vi "MB_TCP_7016_p.vi"(6 "N":i32, 9 "timeouts":T1={"conn_timeout"=1000, "reconn_timeout"=3000, "N attempt max"=3, "t_reset_TTL"=120000, "write_timeout"=10, "read_timeout"=500, "period"=100} {"t_reset_TTL" min=10 max=240000 step=1; "period" min=10 max=100000 step=1; "read_timeout" min=10 max=60000 step=1; "write_timeout" min=1 max=60000 step=1; "N attempt max" min=1 max=5 step=1; "reconn_timeout" min=10 max=240000 step=1; "conn_timeout" min=10 max=240000}, 10 "write enable":bool=TRUE, 11 "stop":bool) -> (0 "error out":errorcluster, 2 "errors":u32, 3 "Z3":u32)   [LabVIEW 2019]
uses:
  NI_modbus_upd/NI_modbus_upd.lvlib
  NI_modbus_upd.llb/MB Modbus Command.ctl
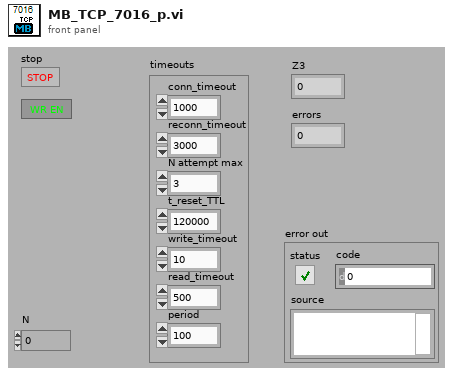
[diagram p1: front panel]
types:
  T1 = cluster{"conn_timeout":i32, "reconn_timeout":u32, "N attempt max":i32, "t_reset_TTL":u32, "write_timeout":i32, "read_timeout":i32, "period":u32}
  T2 = enum16{"Init", "Read", "Read inputs", "Read outputs", "Write", "Write inputs"}
  T3 = enum16{"DI", "DO to write", "DO", "AI", "AO to write", "AO", "DI AI", "DI AO", "DO AI", "DO AO"}
  T4 = enum16{"Start", "Connect", "Write enable", "IP address", "Errors"}
  T5 = typedef "MB Modbus Command.ctl" = cluster{"Function Code":u8, "Starting Address":u16, "Quantity":u16, "Data":u16[], "Discrete":bool[]}
  T6 = cluster{"Transaction ID":u16, "Protocol ID":u16, "Length":u16, "Unit ID":u8}
  T7 = cluster{"Remote IP Address":string, "Remote Port":u16}
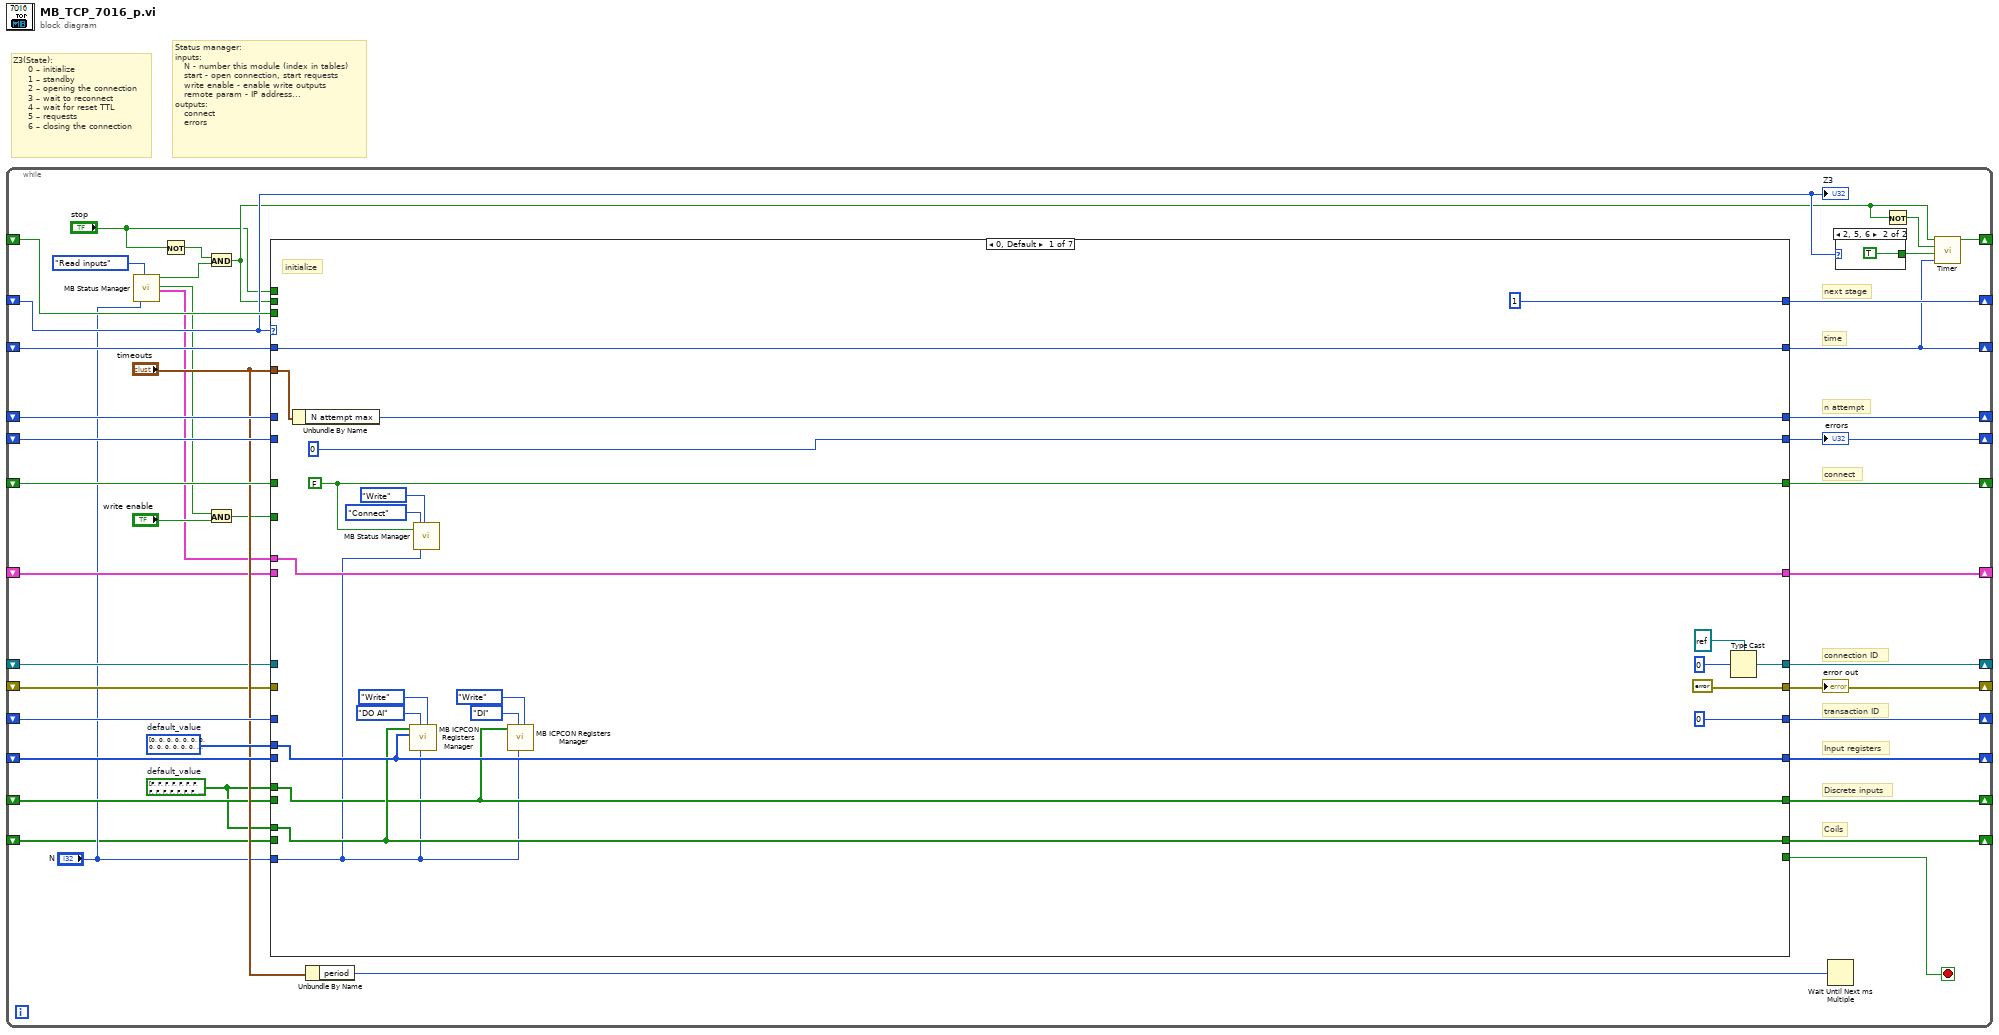
[diagram p0: block diagram]
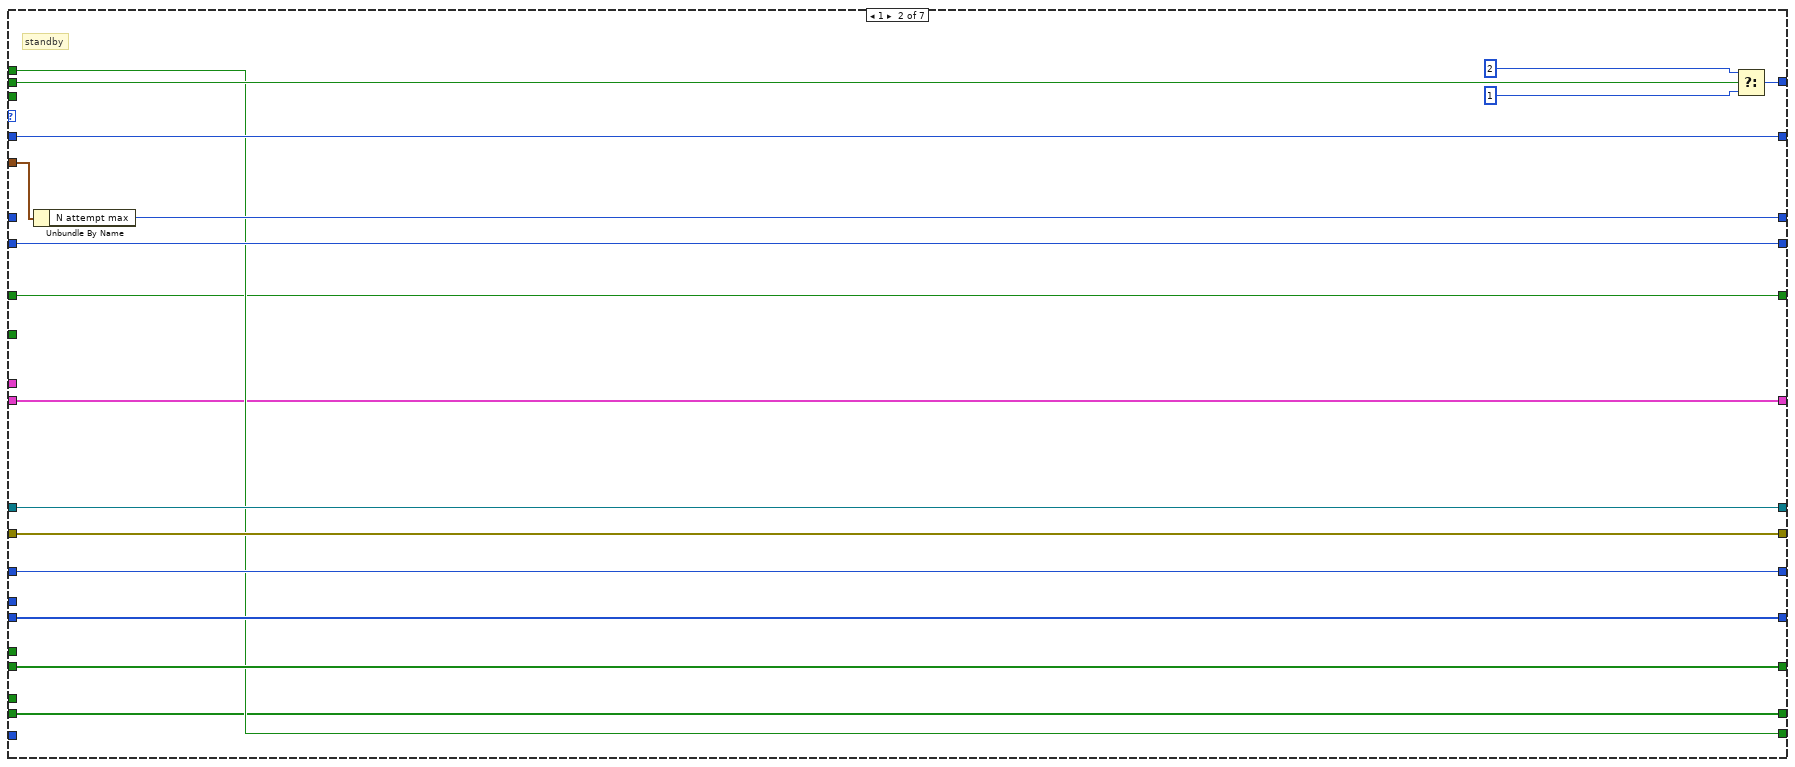
[diagram p2: hidden frame]
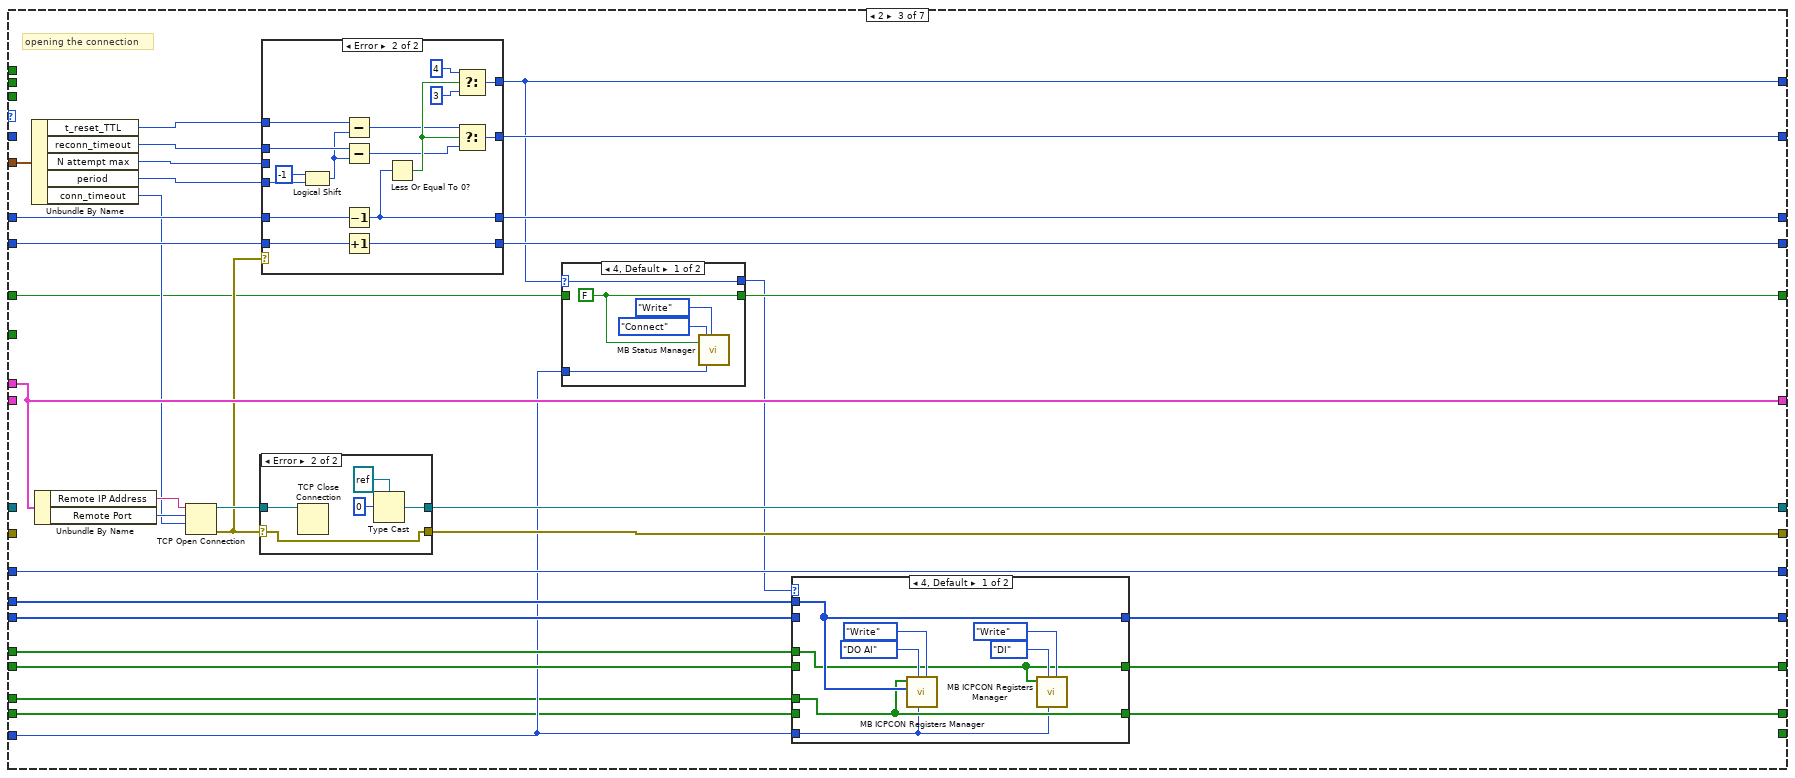
[diagram p3: hidden frame]
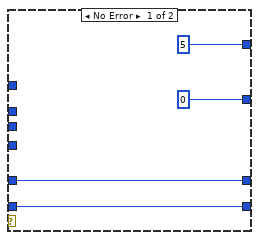
[diagram p7: hidden frame]
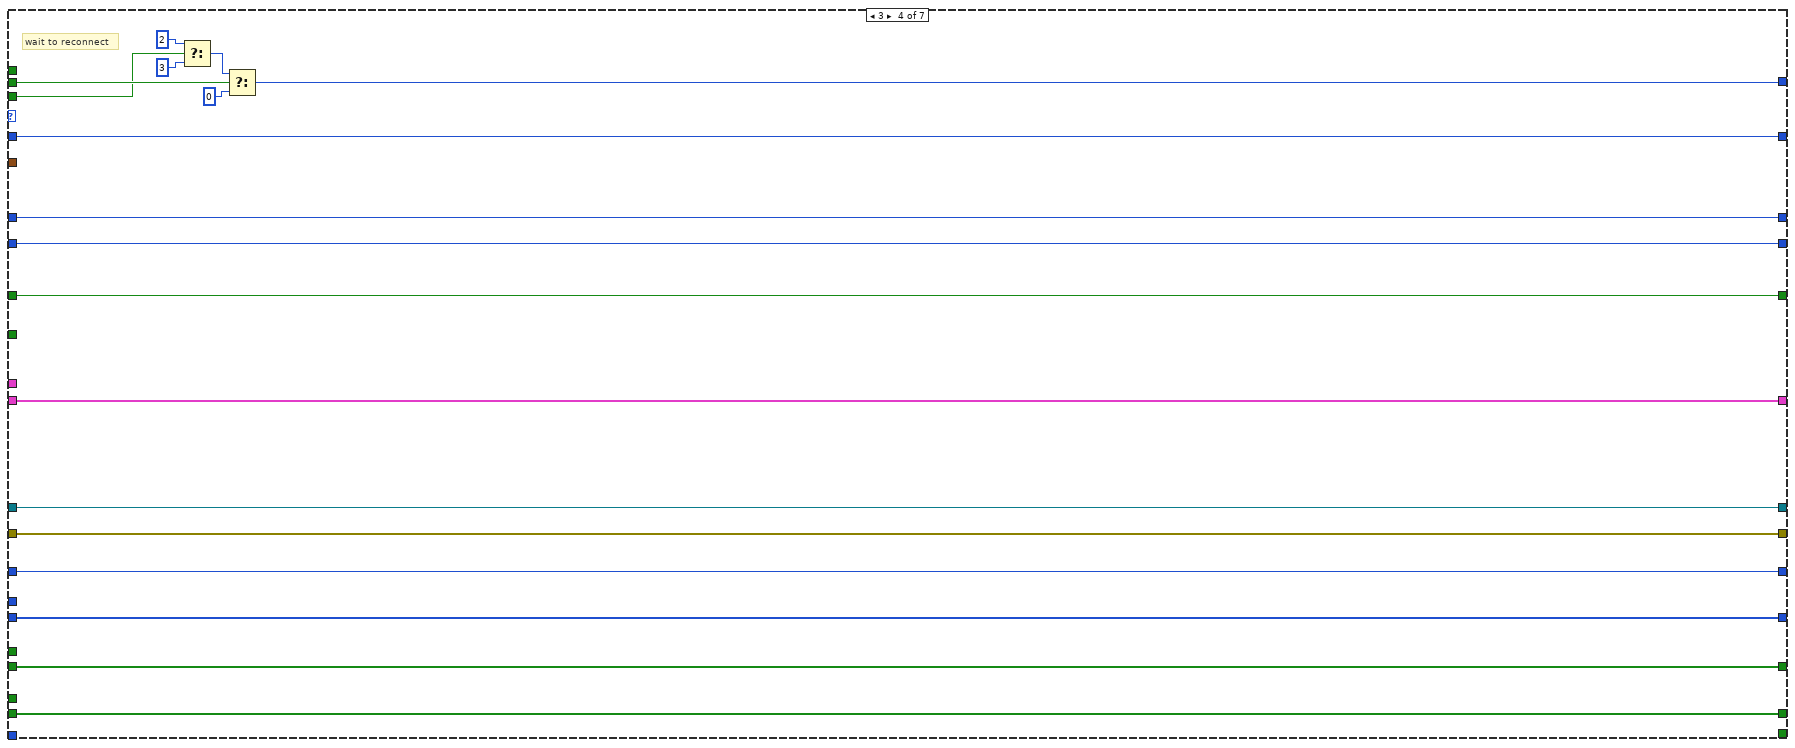
[diagram p8: hidden frame]
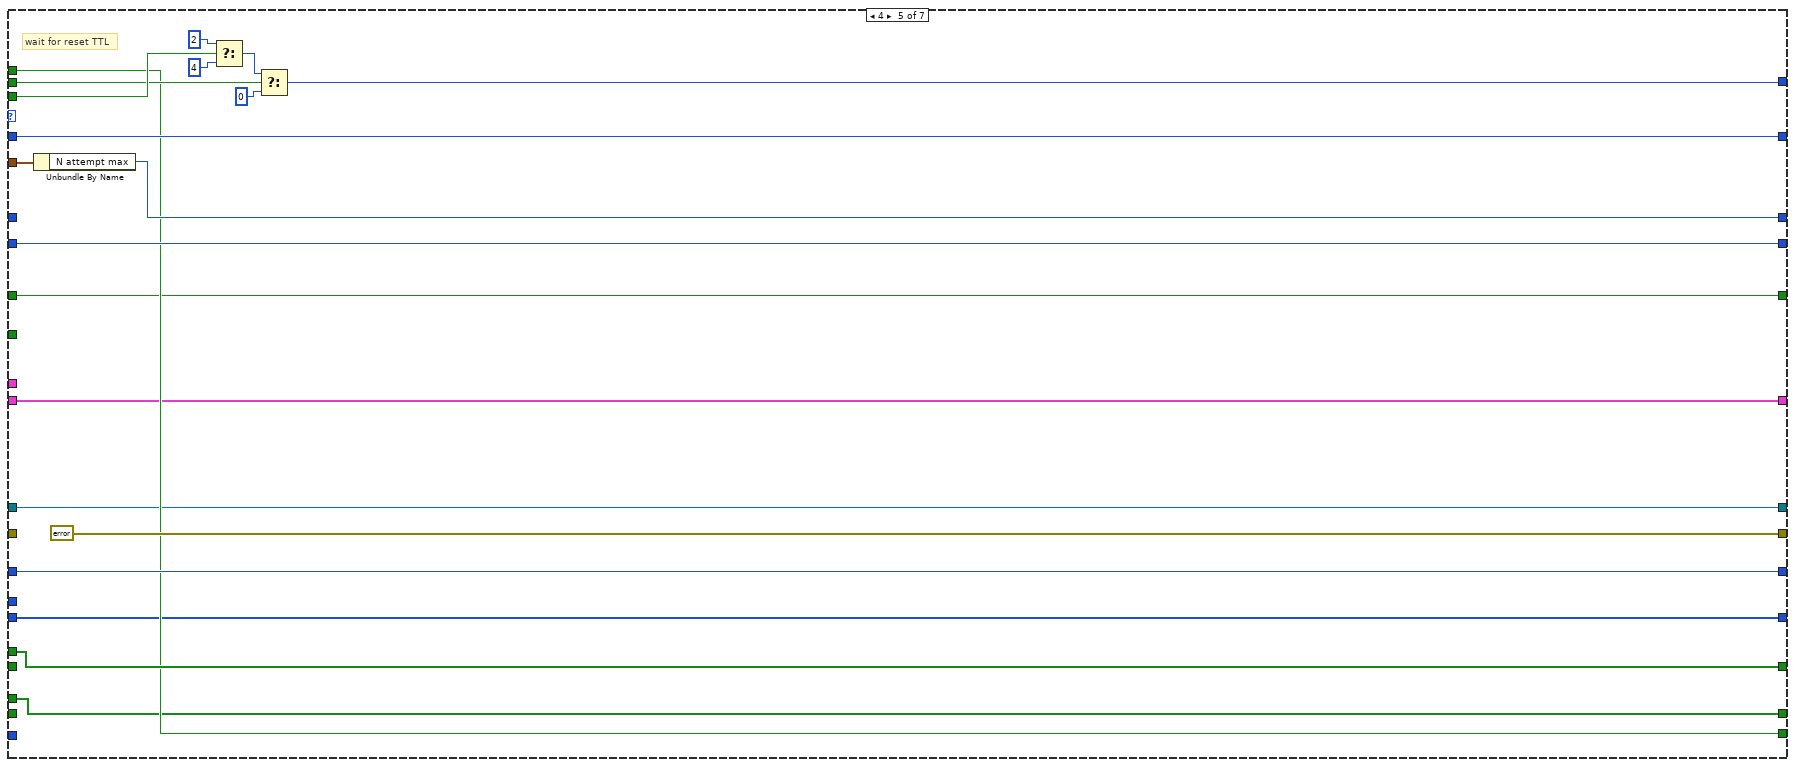
[diagram p9: hidden frame]
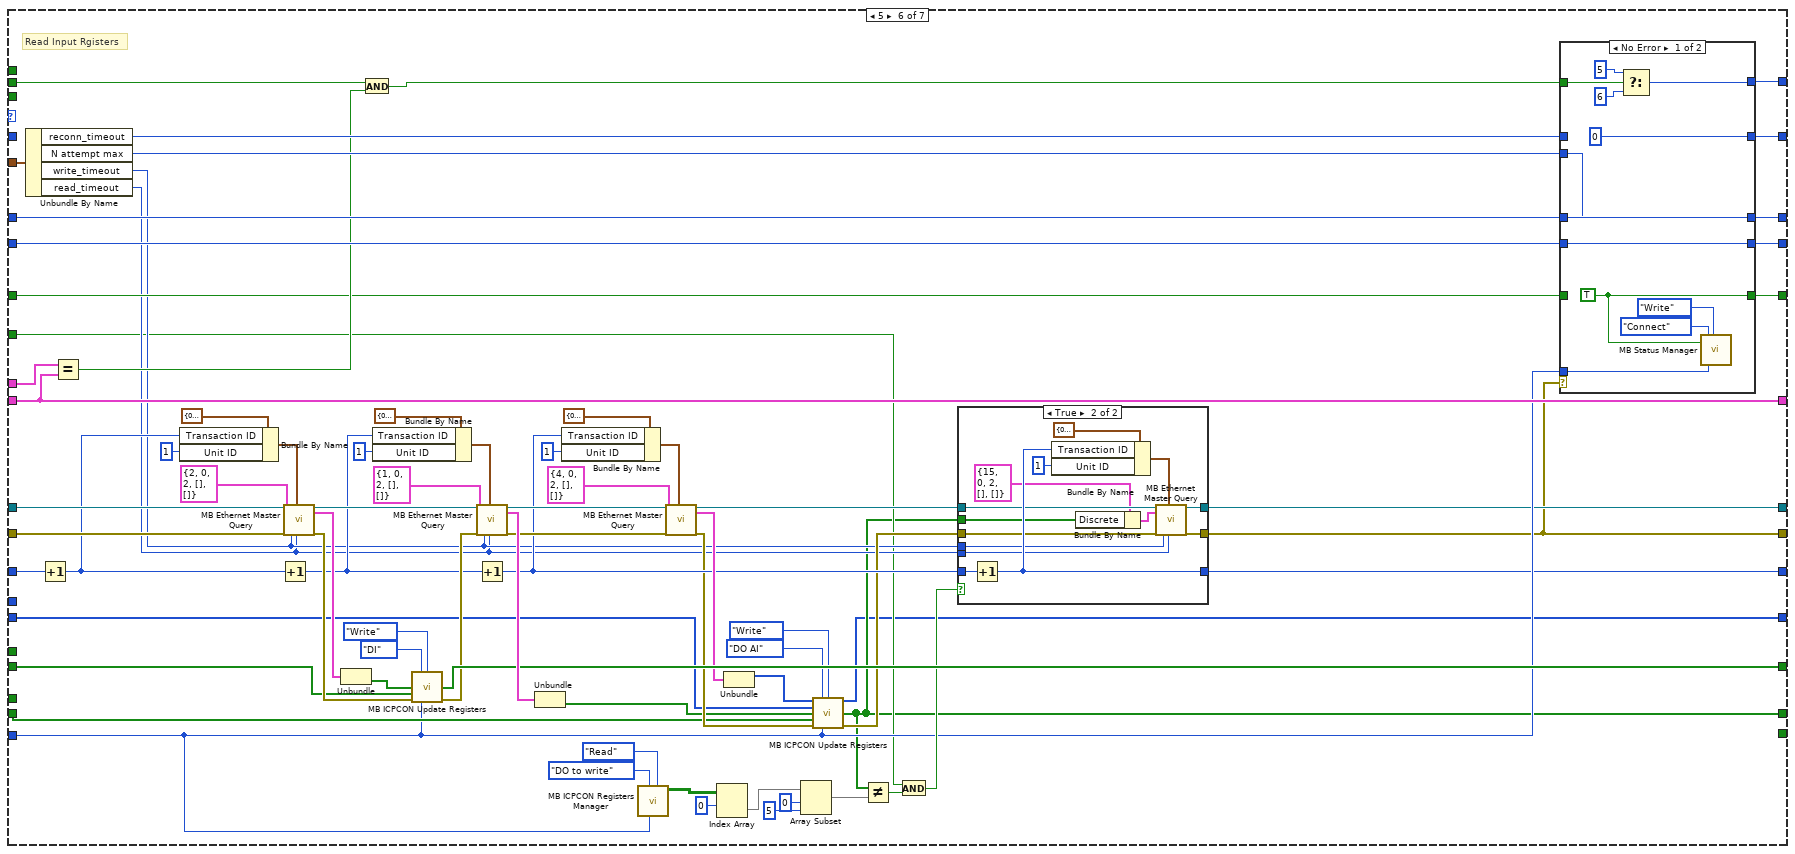
[diagram p10: hidden frame]
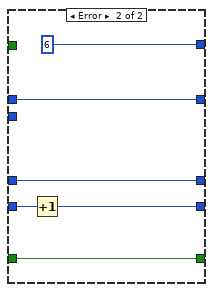
[diagram p12: hidden frame]
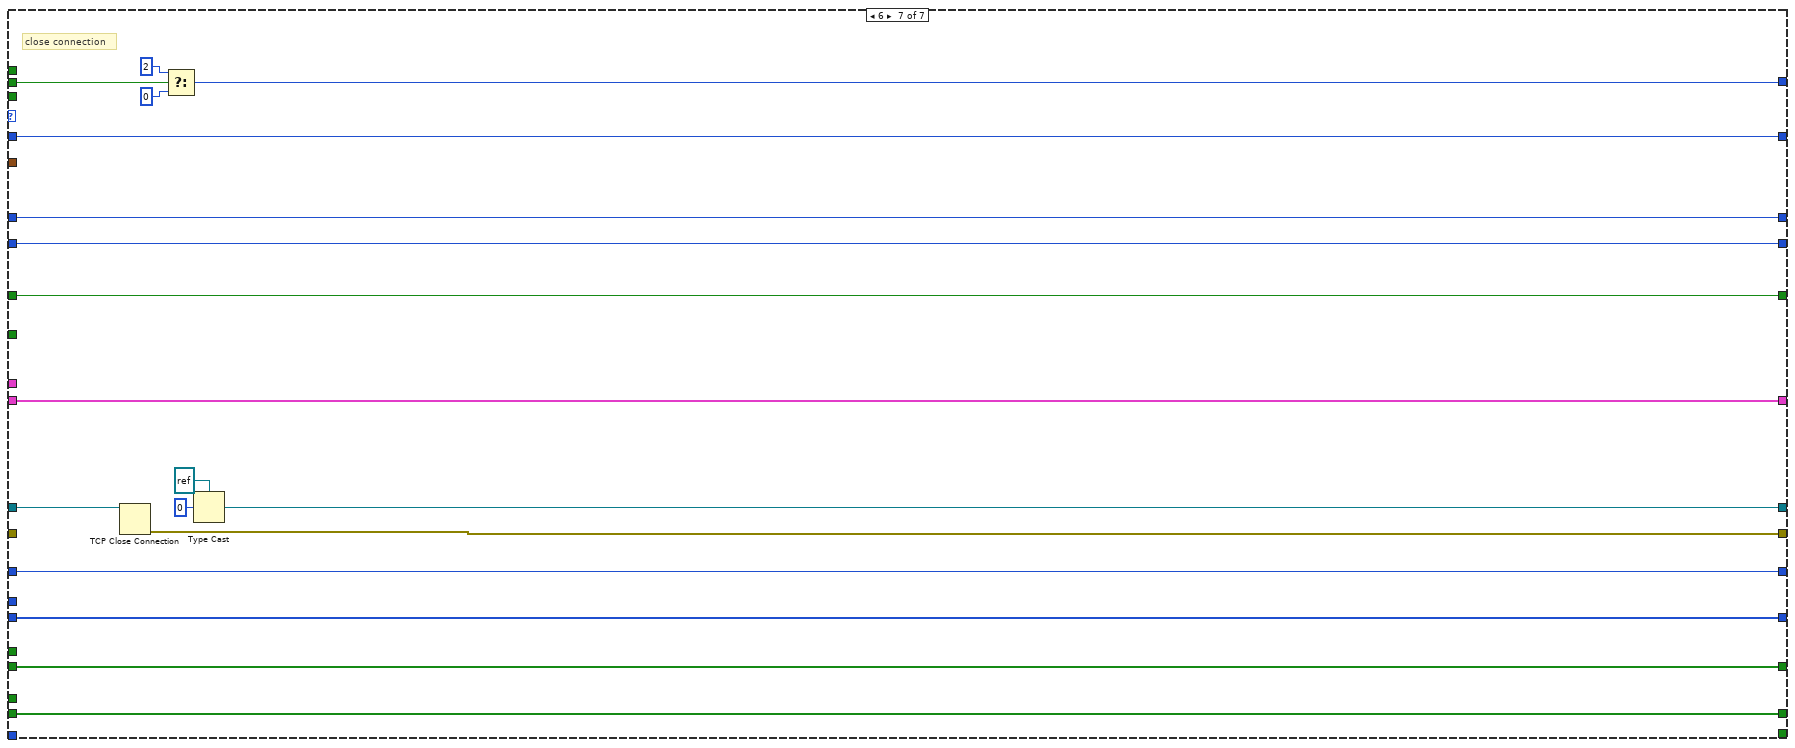
[diagram p13: hidden frame]
diagram:
  # "Status manager:\ninputs:\n   N - number this module (index in tables)\n   start - open connection, start requests\n   write enable - enable write outputs\n   remote param - IP address...\noutputs:\n   connect\n   errors"
  # "Z3(State):\n     0 – initialize \n     1 – standby\n     2 – opening the connection\n     3 – wait to reconnect\n     4 – wait for reset TTL\n     5 – requests\n     6 – closing the connection"
  n1 = while {
    shift-right: [w21] -> _
    shift-left: _ -> [w17]
    shift-right: [w20] -> _
    shift-left: _ -> [w42]
    shift-right: [w41] -> _
    shift-left: _ -> [w39]
    shift-right: [w40] -> _
    shift-left: _ -> [w38]
    shift-right: [w37] -> _
    shift-left: _ -> [w36]
    shift-right: [w35] -> _
    shift-left: _ -> [w22]
    shift-right: [w34] -> _
    shift-left: _ -> [w23]
    shift-right: [w33] -> _
    shift-left: _ -> [w32]
    shift-right: [w31] -> _
    shift-left: _ -> [w30]
    shift-right: [w25] -> _
    shift-left: _ -> [w24]
    shift-right: [w19] -> _
    shift-left: _ -> [w18]
    shift-right: [w10] -> _
    shift-left: _ -> [w9]
    shift-right: [w3] -> _
    shift-left: _ -> [w4]
    stop <- w13 stop-if-true
    w1 = bool[] [FALSE, FALSE, FALSE, FALSE, FALSE, FALSE, FALSE, FALSE, FALSE, FALSE, FALSE, FALSE, FALSE, FALSE, FALSE, FALSE, FALSE, FALSE, FALSE, FALSE, FALSE, FALSE, FALSE, FALSE, FALSE, FALSE, FALSE, FALSE, FALSE, FALSE, FALSE, FALSE]  # default_value
    w29 = u16[] [0, 0, 0, 0, 0, 0, 0, 0, 0, 0, 0, 0, 0, 0, 0, 0, 0, 0, 0, 0]  # default_value
    # "Coils"
    # "Discrete inputs"
    # "Input registers"
    # "connect"
    # "connection ID"
    # "transaction ID"
    # "n attempt"
    # "time"
    # "next stage"
    n2 = call "MB Status Manager.vi"("N"="N", "Function"=T2."Read inputs") -> ("start"=w8:bool, "write enable"=w7:bool, "Remote Param"=w6:T7)  [unwired: 12 in, 3 out]
    n3 = Not(x="stop") -> (.not. x?=w15:bool)
    n4 = And(x=w15, y=w8) -> (x .and. y?=w16:bool)
    n5 = And(x=w7, y="write enable") -> (x .and. y?=w12:bool)
    n6 = case shown="0, Default" w17 {
      tunnel: [w63 w73 w93 w176 w183 w200 w322] -> w35
      tunnel: [errorcluster {"status"=FALSE, "code"=0, "source"=""} ("error out") w72 w91 w175 errorcluster {"status"=FALSE, "code"=0, "source"=""} ("error out") w199 w323] -> w34
      tunnel: w22 -> [_ w73 _ w176 w183 w263 w319]
      tunnel: w23 -> [_ w72 _ w175 _ w262 _]
      tunnel: [w52 w68 w89 w164 w182 w250 w310] -> w37
      tunnel: w36 -> [_ w68 w90 w164 w182 w251 w310]
      tunnel: w6 -> [w55 _ w96 _ _ w257 _]
      tunnel: [w51 w74 w101 w163 w181 w202 w309] -> w31
      tunnel: w30 -> [_ w74 w102 w163 w181 w211 w309]
      tunnel: w32 -> [_ w82 w115 w178 w198 w272 w324]
      tunnel: [u16 0 ("x") w82 w115 w178 w198 w201 w324] -> w33
      tunnel: [w57 w78 w110 w177 w194 w270 w316] -> w41
      tunnel: w39 -> [_ _ w111 w177 _ w270 w316]
      tunnel: [u32 0 ("N attempt max") w81 w113 w174 w197 w269 w321] -> w40
      tunnel: w38 -> [_ w81 w114 w174 w197 w268 w321]
      tunnel: [w59 w80 w107 w173 w196 w265 w320] -> w20
      tunnel: w42 -> [w59 w80 _ w173 w196 _ w320]
      tunnel: "timeouts" -> [w58 w79 w112 _ w195 w271 _]
      tunnel: w16 -> [_ w70 _ w169 w185 w256 w317]
      tunnel: [u32 1 w75 w87 w165 w189 w264 w311] -> w21
      tunnel: w18 -> [_ _ _ w167 w188 _ _]
      tunnel: w29 -> [w51 _ w100 _ _ _ _]
      tunnel: w1 -> [w46 _ w97 _ w186 _ _]
      tunnel: [w46 w71 w98 w166 w186 w240 w314] -> w25
      tunnel: w24 -> [_ w71 w99 w166 _ w213 w314]
      tunnel: "N" -> [w45 _ w88 _ _ w208 _]
      tunnel: "stop" -> [_ w69 _ _ w184 _ _]
      tunnel: [_ w69 _ _ w184 _ _] -> w13
      tunnel: w12 -> [_ _ _ _ _ w204 _]
      tunnel: [w55 w67 w96 w162 w180 w254 w308] -> w10
      tunnel: w9 -> [_ w67 _ w162 w180 w254 w308]
      tunnel: w1 -> [w49 _ w85 _ w179 _ _]
      tunnel: w4 -> [_ w66 w84 w161 _ w209 w307]
      tunnel: [w49 w66 w83 w161 w179 w203 w307] -> w3
      frame 0, Default {
        w52 = FALSE ("connect")
        # "initialize"
        n7 = Unbundle By Name(w58) -> ("N attempt max"=w57:i32)
        n8 = call "MB ICPCON Registers Manager.vi"("Function"=enum16{"Init", "Read", "Write", "Read All"}."Write", "N"=w45, "Table"=T3."DO AI", "Registers In"=w51, "Discrete in"=w49) -> ()  [unwired: 4 in, 3 out]
        n9 = call "MB Status Manager.vi"("connect in"=w52, "Table"=T4."Connect", "N"=w45, "Function"=T2."Write") -> ()  [unwired: 10 in, 6 out]
        n10 = call "MB ICPCON Registers Manager.vi"("Function"=enum16{"Init", "Read", "Write", "Read All"}."Write", "N"=w45, "Table"=T3."DI", "Discrete in"=w46) -> ()  [unwired: 5 in, 3 out]
        n11 = Type Cast(type=refnum<k5> refnum ("connection ID"), x=u32 0) -> (*(type *) &x=w63:refnum<k5>)
      }
      frame 1 {
        # "standby"
        n12 = Unbundle By Name(w79) -> ("N attempt max"=w78:i32)
        n13 = Select(t=u32 2, s=w70, f=u32 1) -> (s? t:f=w75:u32)
      }
      frame 2 {
        # "opening the connection"
        n14 = Unbundle By Name(w112) -> ("t_reset_TTL"=w106:u32, "reconn_timeout"=w108:u32, "N attempt max"=w109:i32, "period"=w103:u32, "conn_timeout"=w95:i32)
        n15 = Unbundle By Name(w96) -> ("Remote IP Address"=w105:string, "Remote Port"=w104:u16)
        n16 = TCP Open Connection(address=w105, remote port or service name=w104, timeout ms (60000)=w95) -> (connection ID=w94:refnum<k5>, error out=w92:errorcluster)  [unwired: 2 in]
        n17 = case shown="Error" w92 {
          selector: w92 -> [w123 w125]
          tunnel: w94 -> [w124 w128]
          tunnel: [w124 w127] -> w93
          tunnel: [w123 w125] -> w91
          frame No Error {
          }
          frame Error {
            n18 = TCP Close Connection(connection ID=w128) -> ()  [unwired: 2 in, 2 out]
            n19 = Type Cast(type=refnum<k5> refnum ("connection ID"), x=u32 0) -> (*(type *) &x=w127:refnum<k5>)
          }
        }
        n20 = case shown="Error" w92 {
          tunnel: w114 -> [w144 w160]
          tunnel: [w144 w159] -> w113
          tunnel: w111 -> [w143 w158]
          tunnel: [w143 w157] -> w110
          tunnel: w109 -> [_ _]
          tunnel: [u32 5 w154] -> w87
          tunnel: w108 -> [_ w153]
          tunnel: [u32 0 w152] -> w107
          tunnel: w106 -> [_ w149]
          tunnel: w103 -> [_ w147]
          frame No Error {
          }
          frame Error {
            n21 = Logical Shift(y=i16 -1, x=w147) -> (x << y=w145:u32)
            n22 = Subtract(x=w149, y=w145) -> (x-y=w148:u32)
            n23 = Subtract(x=w153, y=w145) -> (x-y=w150:u32)
            n24 = Decrement(x=w158) -> (x-1=w157:i32)
            n25 = Increment(x=w160) -> (x+1=w159:u32)
            n26 = Less Or Equal To 0?(x=w157) -> (x <= 0?=w151:bool)
            n27 = Select(t=u32 4, s=w151, f=u32 3) -> (s? t:f=w154:u32)
            n28 = Select(t=w148, s=w151, f=w150) -> (s? t:f=w152:u32)
          }
        }
        n29 = case shown="4, Default" w87 {
          selector: w87 -> [w117 w121]
          tunnel: w88 -> [w118 _]
          tunnel: [w119 w122] -> w89
          tunnel: w90 -> [_ w122]
          tunnel: [w117 w121] -> w86
          frame 4, Default {
            w119 = FALSE ("f")
            n30 = call "MB Status Manager.vi"("connect in"=w119, "Table"=T4."Connect", "N"=w118, "Function"=T2."Write") -> ()  [unwired: 10 in, 6 out]
          }
          frame 3, 5 {
          }
        }
        n31 = case shown="4, Default" w86 {
          tunnel: w88 -> [w131 _]
          tunnel: [w135 w140] -> w101
          tunnel: w102 -> [_ w140]
          tunnel: w100 -> [w135 _]
          tunnel: w99 -> [_ w139]
          tunnel: [w130 w139] -> w98
          tunnel: w97 -> [w130 _]
          tunnel: w85 -> [w134 _]
          tunnel: [w134 w138] -> w83
          tunnel: w84 -> [_ w138]
          frame 4, Default {
            n32 = call "MB ICPCON Registers Manager.vi"("Function"=enum16{"Init", "Read", "Write", "Read All"}."Write", "N"=w131, "Table"=T3."DO AI", "Registers In"=w135, "Discrete in"=w134) -> ()  [unwired: 4 in, 3 out]
            n33 = call "MB ICPCON Registers Manager.vi"("Function"=enum16{"Init", "Read", "Write", "Read All"}."Write", "N"=w131, "Table"=T3."DI", "Discrete in"=w130) -> ()  [unwired: 5 in, 3 out]
          }
          frame 3, 5 {
          }
        }
      }
      frame 3 {
        # "wait to reconnect"
        n34 = Select(t=u32 2, s=w167, f=u32 3) -> (s? t:f=w168:u32)
        n35 = Select(t=w168, s=w169, f=u32 0) -> (s? t:f=w165:u32)
      }
      frame 4 {
        # "wait for reset TTL"
        n36 = Unbundle By Name(w195) -> ("N attempt max"=w194:i32)
        n37 = Select(t=u32 2, s=w188, f=u32 4) -> (s? t:f=w190:u32)
        n38 = Select(t=w190, s=w185, f=u32 0) -> (s? t:f=w189:u32)
      }
      frame 5 {
        # "Read Input Rgisters"
        n39 = Unbundle By Name(w271) -> ("reconn_timeout"=w266:u32, "N attempt max"=w267:i32, "write_timeout"=w206:i32, "read_timeout"=w205:i32)
        n40 = Increment(x=w272) -> (x+1=w244:u16)
        n41 = Equal?(x=w257, y=w254) -> (x = y?=w253:bool)
        n42 = Bundle By Name(cluster=T6 {"Transaction ID"=0, "Protocol ID"=0, "Length"=0, "Unit ID"=0} ("MBAP Header"), "Transaction ID"=w244, "Unit ID"=u8 1) -> (w258:T6)
        n43 = Increment(x=w244) -> (x+1=w228:u16)
        n44 = call "MB Ethernet Master Query.vi"("TCP Connection Refnum in"=w263, "Modbus Command"=T5 {"Function Code"=2, "Starting Address"=0, "Quantity"=2, "Data"=[], "Discrete"=[]}, "error in (no error)"=w262, "Write Timeout"=w206, "MBAP Header"=w258, "Read Timeout"=w205) -> ("TCP Connection Refnum (dup)"=w238:refnum<k5>, "Registers"=w261:cluster{"Registers":u16[], "Discrete":bool[]}, "error out"=w237:errorcluster)  [unwired: 9 in, 2 out]
        n45 = Unbundle(w261) -> ("Discrete"=w214:bool[])  [unwired: 1 out]
        n46 = And(x=w256, y=w253) -> (x .and. y?=w255:bool)
        n47 = Bundle By Name(cluster=T6 {"Transaction ID"=0, "Protocol ID"=0, "Length"=0, "Unit ID"=0} ("MBAP Header"), "Transaction ID"=w228, "Unit ID"=u8 1) -> (w247:T6)
        n48 = call "MB ICPCON Update Registers.vi"("Table"=T3."DI", "Function"=enum16{"Init", "Read", "Write", "Read All"}."Write", "Discrete in"=w214, "Default Discrete in"=w213, "error in (no error)"=w237, "N"=w208) -> ("Discretes"=w240:bool[], "error out"=w236:errorcluster)  [unwired: 7 in, 1 out]
        n49 = call "MB Ethernet Master Query.vi"("TCP Connection Refnum in"=w238, "Modbus Command"=T5 {"Function Code"=1, "Starting Address"=0, "Quantity"=2, "Data"=[], "Discrete"=[]} ("MODBUS Command"), "error in (no error)"=w236, "Write Timeout"=w206, "MBAP Header"=w247, "Read Timeout"=w205) -> ("TCP Connection Refnum (dup)"=w230:refnum<k5>, "Registers"=w242:cluster{"Registers":u16[], "Discrete":bool[]}, "error out"=w227:errorcluster)  [unwired: 9 in, 2 out]
        n50 = Increment(x=w228) -> (x+1=w226:u16)
        n51 = Unbundle(w242) -> ("Discrete"=w210:bool[])  [unwired: 1 out]
        n52 = Bundle By Name(cluster=T6 {"Transaction ID"=0, "Protocol ID"=0, "Length"=0, "Unit ID"=0} ("MBAP Header"), "Transaction ID"=w226, "Unit ID"=u8 1) -> (w231:T6)
        n53 = call "MB ICPCON Registers Manager.vi"("Function"=enum16{"Init", "Read", "Write", "Read All"}."Read", "N"=w208, "Table"=T3."DO to write") -> ("Discretes"=w221:bool[][])  [unwired: 6 in, 2 out]
        n54 = call "MB Ethernet Master Query.vi"("TCP Connection Refnum in"=w230, "Modbus Command"=T5 {"Function Code"=4, "Starting Address"=0, "Quantity"=2, "Data"=[], "Discrete"=[]} ("MODBUS Command"), "error in (no error)"=w227, "MBAP Header"=w231) -> ("TCP Connection Refnum (dup)"=w229:refnum<k5>, "Registers"=w235:cluster{"Registers":u16[], "Discrete":bool[]}, "error out"=w216:errorcluster)  [unwired: 11 in, 2 out]
        n55 = Index Array(array=w221, index (row)=0) -> (element=w219:bool[])  [unwired: 1 in]
        n56 = Unbundle(w235) -> ("Registers"=w212:u16[])  [unwired: 1 out]
        n57 = Array Subset(array=w219, index=0, length=5) -> (w207:bool[])
        n58 = call "MB ICPCON Update Registers.vi"("Registers In"=w212, "Table"=T3."DO AI", "Function"=enum16{"Init", "Read", "Write", "Read All"}."Write", "Default Registers In"=w211, "Discrete in"=w210, "Default Discrete in"=w209, "error in (no error)"=w216, "N"=w208) -> ("Registers"=w202:u16[], "Discretes"=w203:bool[], "error out"=w215:errorcluster)  [unwired: 5 in]
        n59 = Not Equal?(x=w203, y=w207) -> (x != y?=w241:bool)
        n60 = And(x=w204, y=w241) -> (x .and. y?=w239:bool)
        n61 = case shown="True" w239 {
          tunnel: w205 -> [_ w280]
          tunnel: w206 -> [_ w279]
          tunnel: w226 -> [w274 w287]
          tunnel: [w274 w286] -> w201
          tunnel: w215 -> [w273 w284]
          tunnel: [w273 w283] -> w199
          tunnel: w229 -> [w275 w282]
          tunnel: [w275 w281] -> w200
          tunnel: w203 -> [_ w276]
          frame False {
          }
          frame True {
            n62 = Increment(x=w287) -> (x+1=w286:u16)
            n63 = Bundle By Name(cluster=T6 {"Transaction ID"=0, "Protocol ID"=0, "Length"=0, "Unit ID"=0} ("MBAP Header"), "Transaction ID"=w286, "Unit ID"=u8 1) -> (w288:T6)
            n64 = Bundle By Name(cluster=T5 {"Function Code"=15, "Starting Address"=0, "Quantity"=2, "Data"=[], "Discrete"=[]} ("MODBUS Command"), "Discrete"=w276) -> (w277:T5)
            n65 = call "MB Ethernet Master Query.vi"("TCP Connection Refnum in"=w282, "Modbus Command"=w277, "error in (no error)"=w284, "Write Timeout"=w279, "MBAP Header"=w288, "Read Timeout"=w280) -> ("TCP Connection Refnum (dup)"=w281:refnum<k5>, "error out"=w283:errorcluster)  [unwired: 9 in, 3 out]
          }
        }
        n66 = case shown="No Error" w199 {
          tunnel: w268 -> [w294 w306]
          tunnel: [w294 w305] -> w269
          tunnel: [w296 u32 6] -> w264
          tunnel: w270 -> [_ w303]
          tunnel: w267 -> [w300 _]
          tunnel: [w300 w303] -> _
          tunnel: w266 -> [_ w302]
          tunnel: [u32 0 w302] -> w265
          tunnel: w255 -> [w295 _]
          tunnel: w251 -> [_ w301]
          tunnel: [w292 w301] -> w250
          tunnel: w208 -> [w291 _]
          frame No Error {
            w292 = TRUE ("f")
            n67 = Select(t=u32 5, s=w295, f=u32 6) -> (s? t:f=w296:u32)
            n68 = call "MB Status Manager.vi"("connect in"=w292, "Table"=T4."Connect", "N"=w291, "Function"=T2."Write") -> ()  [unwired: 10 in, 6 out]
          }
          frame Error {
            n69 = Increment(x=w306) -> (x+1=w305:u32)
          }
        }
      }
      frame 6 {
        # "close connection"
        n70 = TCP Close Connection(connection ID=w319) -> (error out=w323:errorcluster)  [unwired: 2 in, 1 out]
        n71 = Select(t=u32 2, s=w317, f=u32 0) -> (s? t:f=w311:u32)
        n72 = Type Cast(type=refnum<k5> refnum ("connection ID"), x=u32 0) -> (*(type *) &x=w322:refnum<k5>)
      }
    }
    "error out" <- w34
    "errors" <- w40
    n73 = Unbundle By Name("timeouts") -> ("period"=w27:u32)
    n74 = Wait Until Next ms Multiple(millisecond multiple=w27) -> ()  [unwired: 1 out]
    n75 = case shown="2, 5, 6" w17 {
      tunnel: [_ TRUE] -> w26
      frame 0, Default {
      }
      frame 2, 5, 6 {
      }
    }
    n76 = Not(x=w16) -> (.not. x?=w43:bool)
    n77 = call "Timer.vi"("ms"=w20, "Load (F)"=w26, "Reset (F)"=w43, "Start (T)"=w16) -> ("End"=w19:bool)  [unwired: 5 in, 1 out]
    "Z3" <- w17
  }
